vi "UR3 Animation.vi"() -> ()   [LabVIEW 2024]
uses:
  <vilib>/Analysis/Matrix/Datatypes/RealMatrix.ctl
  <vilib>/Utility/miscctls.llb/LV3DPointTypeDef.ctl
  <vilib>/Analysis/Matrix/NI_Matrix.lvlib
panel:
  in  "Threshold":dbl=1e-05
  in  "Max Iterations":i32=100
  in  "intermediate points":i32=100
  out "Number of iterations":i32[](graph)
  out "end pose":T1
  out "starting pose":T1=[[1.0, 0.0, 0.0, 0.0], [0.0, 6.123233995736766e-17, 1.0, 0.0], [0.0, -1.0, 6.123233995736766e-17, 0.0], [0.0, 0.0, 0.0, 1.0]] format="%#_2g"
  out "qe (deg)":sgl[](array[numeric])
  out "3D Picture":refnum<vi>(3d-picture)
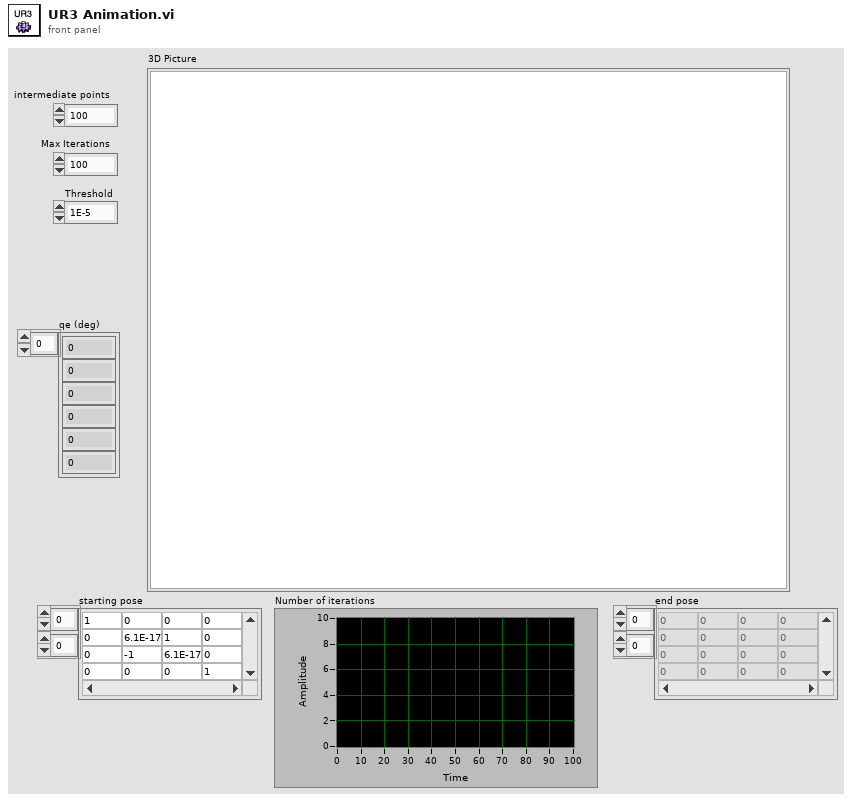
[diagram p1: front panel]
types:
  T1 = typedef "NI_Matrix.lvlib/RealMatrix.ctl" = dbl[][]
  T2 = typedef "LV3DPointTypeDef.ctl" = cluster{"X":sgl, "Y":sgl, "Z":sgl}
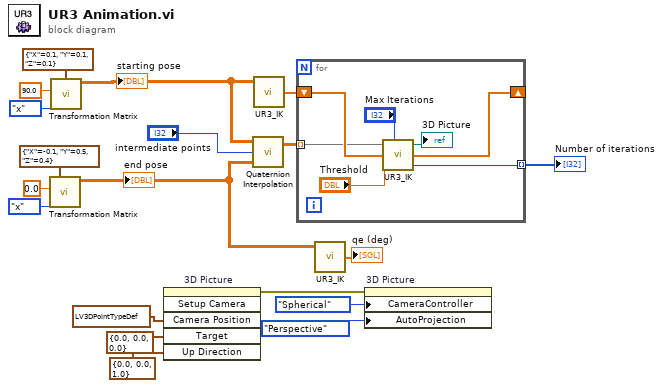
[diagram p0: block diagram]
diagram:
  n1 = call <userlib>:"Transformation Matrix.vi"("Axis"=enum16{"x", "y", "z"}."x", "Angle (degrees)"=0.0, "Translation"=cluster{"X":dbl, "Y":dbl, "Z":dbl} {"X"=-0.1, "Y"=0.5, "Z"=0.4}) -> ("Transformation Matrix"=w4:T1)  [unwired: 8 in]
  "end pose" <- w4
  n2 = call <userlib>:"Transformation Matrix.vi"("Axis"=enum16{"x", "y", "z"}."x", "Angle (degrees)"=90.0, "Translation"=cluster{"X":dbl, "Y":dbl, "Z":dbl} {"X"=0.1, "Y"=0.1, "Z"=0.1}) -> ("Transformation Matrix"=w5:T1)  [unwired: 8 in]
  "starting pose" <- w5
  n3 = invoke on="3D Picture" class="SceneGraphDisp (strict)" method="Setup Camera"("Camera Position"=T2 {"X"=0.4, "Y"=1.5, "Z"=0.1}, "Target"=cluster{"X":sgl, "Y":sgl, "Z":sgl} {"X"=0.0, "Y"=0.0, "Z"=0.0}, "Up Direction"=cluster{"X":sgl, "Y":sgl, "Z":sgl} {"X"=0.0, "Y"=0.0, "Z"=1.0}) -> (error out=w19:errorcluster)  [unwired: 3 in, 5 out]
  n4 = call <userlib>:"Quaternion Interpolation.vi"("end pose"=w4, "intermediate points"="intermediate points", "start pose"=w5) -> ("interpolations"=w9:dbl[][][])  [unwired: 1 in]
  n5 = call <userlib>:"UR3_IK.vi"("Transformation Matrix"=w5) -> ("q (deg)"=w3:dbl[])  [unwired: 4 in, 2 out]
  n6 = for {
    tunnel: w9 -> [w25] mode=indexing
    shift-right: [w23] -> _
    shift-left: w3 -> [w26]
    tunnel: [w22] -> w1 mode=indexing
    n7 = call <userlib>:"UR3_IK.vi"("Transformation Matrix"=w25, "Max Iterations"="Max Iterations", "guess (deg)"=w26, "Threshold"="Threshold") -> ("3D Picture"=→"3D Picture":refnum<vi>, "q (deg)"=w23:dbl[], "iterations"=w22:i32)  [unwired: 1 in]
  }
  "Number of iterations" <- w1
  n8 = call <userlib>:"UR3_IK.vi"("Transformation Matrix"=w4) -> ("q (deg)"=→"qe (deg)":dbl[])  [unwired: 4 in, 2 out]
  n9 = property on="3D Picture" class="SceneGraphDisp (strict)"(error in=w19, "CameraController"=enum16{"None", "Spherical", "Flying"}."Spherical" ("Camera Controller"), "AutoProjection"=enum16{"None", "Perspective", "Orthographic"}."Perspective" ("Auto Projection Mode")) -> ()  [unwired: 1 in, 2 out]
